vi "ExampleDC.vi"() -> ()   [LabVIEW 2024]
uses:
  DCMotor/DCMotor.lvclass
  <vilib>/MakerHub/LINX/LMH-LINX.lvlib
  <vilib>/MakerHub/LINX/Public/Utilities/Open Local.vi
panel:
  in  "GO":bool
  in  "Enum":enum16{"Bacward", "Forward", "Release"}(ring)=enum."Forward"
  out "Error Out":errorcluster
  in  "stop":bool
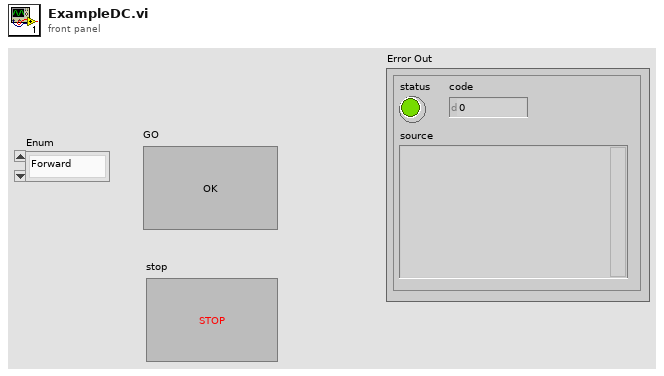
[diagram p1: front panel]
types:
  T1 = typedef "LMH-LINX.lvlib/LINX Ref.ctl" = cluster{"IO":T2, "Interface":T3, "LINX Device Config":T4}
  T2 = typedef "LMH-LINX.lvlib/Platform.ctl" = enum16{"Remote", "Local"}
  T3 = typedef "LMH-LINX.lvlib/Interface.ctl" = enum16{"Serial", "TCP"}
  T4 = typedef "LMH-LINX.lvlib/Device.lvlib/LINX Device Config.ctl" = cluster{"Interface":T3, "COM Port":refnum<visa-resource-name>, "TCP Configuration":T5, "Device Family":u8, "Device ID":u8, "Device Name":string, "TCP Ref":refnum<k5>, "Channels":T6}
  T5 = typedef "LMH-LINX.lvlib/Device.lvlib/TCP Config.ctl" = cluster{"IP Address":string, "Port":u16}
  T6 = typedef "LMH-LINX.lvlib/Channels.ctl" = cluster{"DI":u8[], "DO":u8[], "AI":u8[], "AO":u8[], "PWM":u8[], "QE":u8[], "UART":u8[], "I2C 2":u8[], "SPI":u8[], "CAN":u8[], "Servo":u8[], "AI Ref (V)":dbl, "AI Resolution (Bits)":u8, "AO Ref (V)":dbl, "AO Resolution (Bits)":u8}
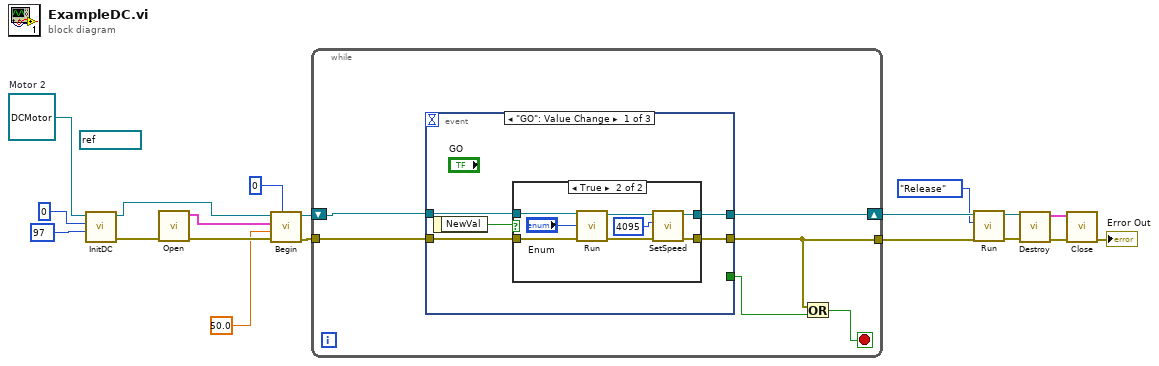
[diagram p0: block diagram]
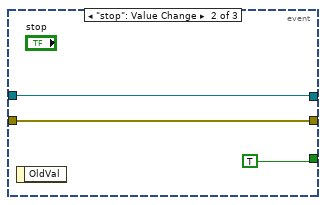
[diagram p3: hidden frame]
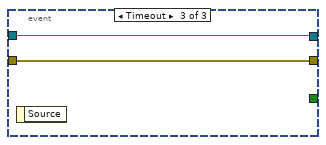
[diagram p4: hidden frame]
diagram:
  (unwired) refnum<visa-resource-name> "COM4" ("Serial Port")
  w17 = refnum<class "DCMotor.lvclass"> refnum  # Motor 2
  n1 = call "InitDC.vi"("_addr"=u8 97, "Motornum"=u8 0, "DCMotor in"=w17) -> ("error out"=w16:errorcluster, "DCMotor out"=w13:refnum<class "DCMotor.lvclass">)  [unwired: 7 in]
  n2 = call-poly <vilib>:"Open.vi"("Error In"=w16) -> ("Error Out"=w15:errorcluster, "LINX Resource"=w14:T1)  [unwired: 8 in, 1 out]
  n3 = call-dynamic "Begin.vi"("I2C Chanel(1)"=0, "error in (no error)"=w15, "_freq"=sgl 50.0, "LINX Resource"=w14, "DCMotor in"=w13) -> ("error out"=w11:errorcluster, "DCMotor out"=w10:refnum<class "DCMotor.lvclass">)  [unwired: 4 in, 1 out]
  n4 = while {
    tunnel: w11 -> [w25]
    tunnel: [w22] -> w4
    shift-right: [w21] -> w5
    shift-left: w10 -> [w24]
    stop <- w23 stop-if-true
    n5 = event shown="[0] \"GO\": Value Change" {
      selector: _ -> [_ _ _]
      dyn-events: _ -> [_ _ _]
      timeout: _ -> [_ _ _]
      tunnel: w25 -> [w30 w43 w44]
      tunnel: w24 -> [w29 w42 w45]
      tunnel: [w28 w43 w44] -> w22
      tunnel: [w27 w42 w45] -> w21
      tunnel: [_ TRUE _] -> w20
      event "GO": Value Change {
        n6 = event-data() -> ("NewVal"=w26:bool)  [unwired: 1 in]
        n7 = case shown="True" w26 {
          tunnel: w30 -> [w31 w40]
          tunnel: w29 -> [w32 w39]
          tunnel: [w31 w38] -> w28
          tunnel: [w32 w37] -> w27
          frame False {
          }
          frame True {
            n8 = call "Run.vi"("error in (no error)"=w40, "Enum"="Enum", "DCMotor in"=w39) -> ("error out"=w36:errorcluster, "DCMotor out"=w35:refnum<class "DCMotor.lvclass">)  [unwired: 7 in]
            n9 = call "SetSpeed.vi"("error in (no error)"=w36, "Speed(0..4095)"=u16 4095 ("Speed(0..255)"), "DCMotor in"=w35) -> ("error out"=w38:errorcluster, "DCMotor out"=w37:refnum<class "DCMotor.lvclass">)  [unwired: 7 in]
          }
        }
      }
      event "stop": Value Change {
        n10 = event-data() -> ()  [unwired: 1 in, 1 out]
      }
      event Timeout {
        n11 = event-data() -> ()  [unwired: 1 in, 1 out]
      }
    }
    n12 = Or(x=w22, y=w20) -> (x .or. y?=w23:bool)
  }
  n13 = call "Run.vi"("error in (no error)"=w4, "Enum"=enum16{"Bacward", "Forward", "Release"}."Release", "DCMotor in"=w5) -> ("error out"=w3:errorcluster, "DCMotor out"=w2:refnum<class "DCMotor.lvclass">)  [unwired: 7 in]
  n14 = call-dynamic "Destroy.vi"("error in (no error)"=w3, "DCMotor in"=w2) -> ("error out"=w9:errorcluster, "LINX Resource"=w8:T1)  [unwired: 8 in]
  n15 = call <vilib>:"Close.vi"("Error In"=w9, "LINX Resource"=w8) -> ("Error Out"=→"Error Out":errorcluster)  [unwired: 9 in]
